vi "appendRawDataToWaveformTest.vi"(6 "Czułości [V/g]":dbl[](array[numeric]), 8 "ErrorIn":errorcluster, 9 "Tacho signal In":waveform(dbl), 10 "RawAccData":waveform(dbl)[](array[waveform]), 11 "AccelerationDataIn":waveform(dbl)[](array[waveform])=[{"t0"=timestamp(0 s since 1904-01-01), "dt"=0.0, "Y"=[]}, {"t0"=timestamp(0 s since 1904-01-01), "dt"=0.0, "Y"=[]}, {"t0"=timestamp(0 s since 1904-01-01), "dt"=0.0, "Y"=[]}]) -> (0 "ErrorOut":errorcluster, 2 "Tacho signal Out":waveform(dbl), 3 "AccelerationDataOut":waveform(dbl)[](array[waveform]))   [LabVIEW 2019]
uses:
  <vilib>/Waveform/WDTOps.llb/WDT Append Waveforms DBL.vi
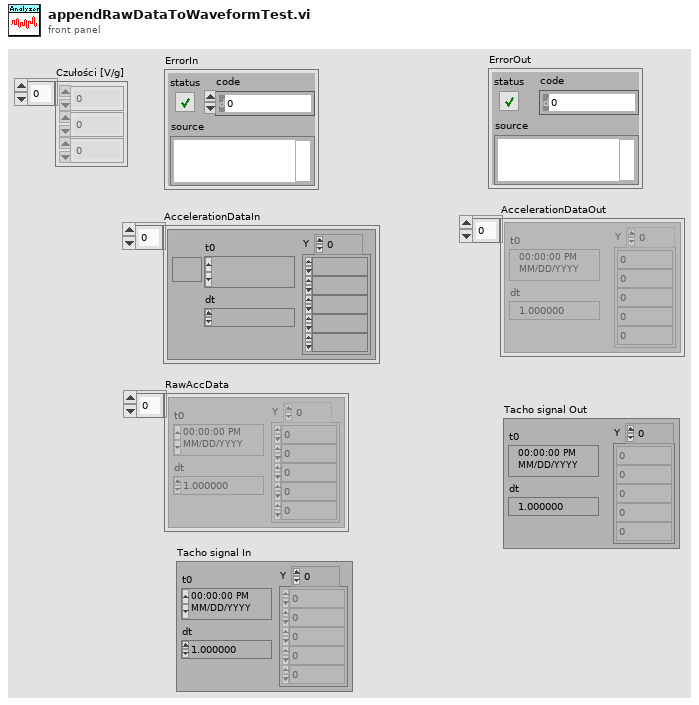
[diagram p1: front panel]
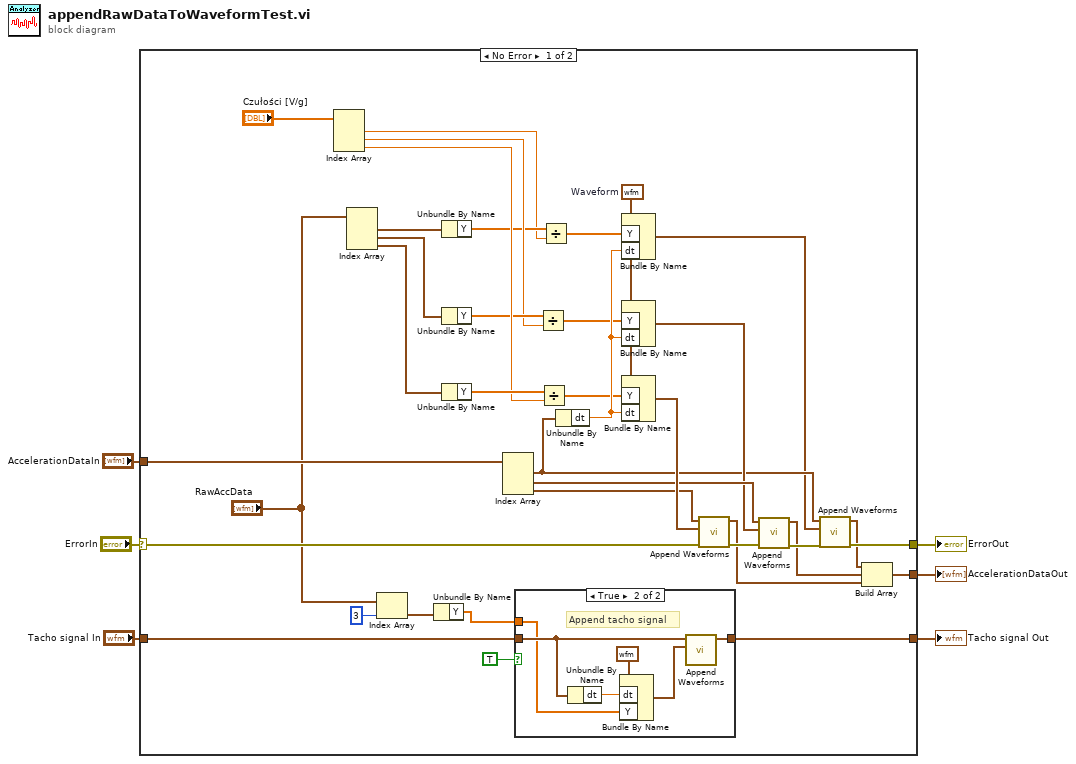
[diagram p0: block diagram]
diagram:
  n1 = case shown="No Error" "ErrorIn" {
    selector: "ErrorIn" -> [w26 w53]
    tunnel: [w37 w53] -> w5
    tunnel: "AccelerationDataIn" -> [w32 w51]
    tunnel: [w31 w51] -> w1
    tunnel: "Tacho signal In" -> [w28 w52]
    tunnel: [w24 w52] -> w2
    frame No Error {
      w43 = waveform(dbl) {"t0"=timestamp(0 s since 1904-01-01), "dt"=0.0, "Y"=[]}  # Waveform
      n2 = Index Array(array="Czułości [V/g]") -> (element #1=w7:dbl, element #2=w9:dbl, element #3=w11:dbl)  [unwired: 3 in]
      n3 = Index Array(array="RawAccData") -> (element #1=w21:waveform(dbl), element #2=w20:waveform(dbl), element #3=w19:waveform(dbl))  [unwired: 3 in]
      n4 = Index Array(array="RawAccData", index=3 ("disabled index (col)")) -> (element=w18:waveform(dbl))
      n5 = Unbundle By Name(w18) -> ("Y"=w17:dbl[])
      n6 = Unbundle By Name(w21) -> ("Y"=w8:dbl[])
      n7 = Unbundle By Name(w20) -> ("Y"=w10:dbl[])
      n8 = Unbundle By Name(w19) -> ("Y"=w12:dbl[])
      n9 = Index Array(array=w32) -> (element #1=w30:waveform(dbl), element #2=w40:waveform(dbl), element #3=w41:waveform(dbl))  [unwired: 3 in]
      n10 = case shown="True" TRUE {
        tunnel: w28 -> [w44 w47]
        tunnel: [w44 w46] -> w24
        tunnel: w17 -> [_ w45]
        frame False {
        }
        frame True {
          # "Append tacho signal"
          n11 = Unbundle By Name(w47) -> ("dt"=w49:dbl)
          n12 = Bundle By Name(cluster=waveform(dbl) {"t0"=timestamp(0 s since 1904-01-01), "dt"=0.0, "Y"=[]} ("analog tacho signal"), "dt"=w49, "Y"=w45) -> (w48:waveform(dbl))
          n13 = call-poly <vilib>:"Append Waveforms.vi"("waveform B"=w48, "waveform A"=w47) -> ("waveform out"=w46:waveform(dbl))  [unwired: 8 in, 1 out]
        }
      }
      n14 = Divide(x=w10, y=w9) -> (x/y=w14:dbl[])
      n15 = Divide(x=w12, y=w11) -> (x/y=w13:dbl[])
      n16 = Divide(x=w8, y=w7) -> (x/y=w15:dbl[])
      n17 = Unbundle By Name(w30) -> ("dt"=w29:dbl)
      n18 = Bundle By Name(cluster=w43, "Y"=w15, "dt"=w29) -> (w23:waveform(dbl))
      n19 = Bundle By Name(cluster=w43, "Y"=w14, "dt"=w29) -> (w36:waveform(dbl))
      n20 = Bundle By Name(cluster=w43, "Y"=w13, "dt"=w29) -> (w42:waveform(dbl))
      n21 = call-poly <vilib>:"Append Waveforms.vi"("error in (no error)"=w26, "waveform B"=w42, "waveform A"=w41) -> ("error out"=w39:errorcluster, "waveform out"=w35:waveform(dbl))  [unwired: 7 in]
      n22 = call-poly <vilib>:"Append Waveforms.vi"("error in (no error)"=w39, "waveform B"=w36, "waveform A"=w40) -> ("error out"=w38:errorcluster, "waveform out"=w34:waveform(dbl))  [unwired: 7 in]
      n23 = call-poly <vilib>:"Append Waveforms.vi"("error in (no error)"=w38, "waveform B"=w23, "waveform A"=w30) -> ("error out"=w37:errorcluster, "waveform out"=w33:waveform(dbl))  [unwired: 7 in]
      n24 = Build Array(w33, w34, w35) -> (w31:waveform(dbl)[])
    }
    frame Error {
    }
  }
  "ErrorOut" <- w5
  "AccelerationDataOut" <- w1
  "Tacho signal Out" <- w2
